vi "Configure Power Measurement Parameters.vi"(7 "Step Length (576.9230769E-6)":dbl=0.0005769230769 format="%^.7e", 8 "error in (no error)":errorcluster, 9 "Measurement Length (300.0E-6)":dbl=0.0003 format="%^.3e", 10 "Instance (1)":i32=1 format="%.0g", 11 "VISA resource name":refnum<visa-resource-name>) -> (0 "error out":errorcluster, 3 "VISA resource name out":refnum<visa-resource-name>)   [LabVIEW 2020, in "Rohde&Schwarz CMXP GPRF.lvlib"]
doc: "Configures power measurement parameters.\n\nAttributes:\nRSCMXPGPRF_ATTR_POWER_MEASUREMENT_MEASUREMENT_LENGTH\nRSCMXPGPRF_ATTR_POWER_MEASUREMENT_STEP_LENGTH\n\nRemote-control commands:\nCONFigure:GPRF:MEAS<i>:POWer:MLENgth\nCONFigure:GPRF:MEAS<i>:POWer:SLENgth"
uses:
  <instrlib>/Rohde&Schwarz CMXP GPRF/Rohde&Schwarz CMXP GPRF.lvlib
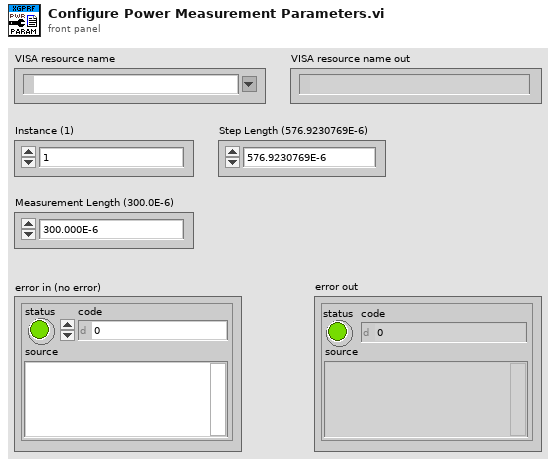
[diagram p1: front panel]
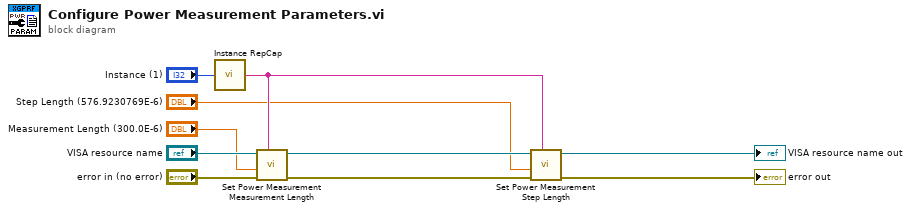
[diagram p0: block diagram]
diagram:
  n1 = call <instrlib>:"Instance RepCap.vi"("Instance in"="Instance (1)") -> ("Instance out"=w9:string)
  n2 = call "Set Power Measurement Measurement Length"("Repeated Capabilities"=w9, "error in (no error)"="error in (no error)", "Power Measurement Measurement Length (0.0)"="Measurement Length (300.0E-6)", "instrument handle"="VISA resource name") -> ("error out"=w7:errorcluster, "instrument handle out"=w8:refnum<visa-resource-name>)  [unwired: 6 in]
  n3 = call "Set Power Measurement Step Length"("Repeated Capabilities"=w9, "error in (no error)"=w7, "Power Measurement Step Length (0.0)"="Step Length (576.9230769E-6)", "instrument handle"=w8) -> ("error out"=→"error out":errorcluster, "instrument handle out"=→"VISA resource name out":refnum<visa-resource-name>)  [unwired: 6 in]
